vi "UI_FP size and position.vi"(4 "Close Ref? (T) In":bool=TRUE, 6 "Move Window (f) In":bool, 7 "FP Origin (0,0) In":cluster{"Horizontal":i16, "Vertical":i16}, 8 "Error In":errorcluster, 9 "Window Size(No Resize) In":cluster{"Width":i16, "Height":i16}, 10 "Window Origin (0,0) In":cluster{"Left":i16, "Top":i16}, 11 "Vi Ref (this Vi) In":refnum<vi>) -> (0 "Error Out":errorcluster, 3 "Dup Ref Out":refnum<vi>)   [LabVIEW 2009]
doc: "Sets VI Front Panel to specified position and size"
panel:
  in  "Set Values":bool
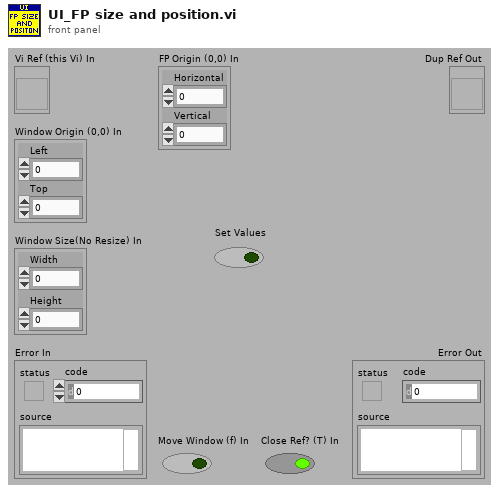
[diagram p1: front panel]
types:
  T1 = typedef "LVRectTypeDef.ctl" = cluster{"left":i16, "top":i16, "right":i16, "bottom":i16}
  T2 = typedef "LVPointTypeDef.ctl" = cluster{"Horizontal":i16, "Vertical":i16}
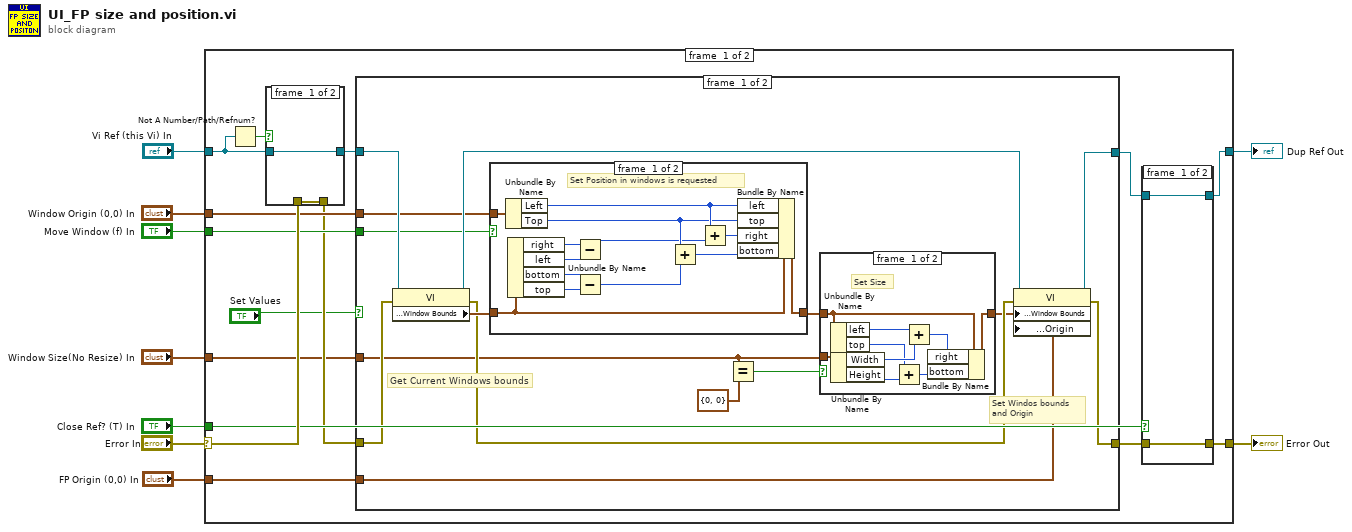
[diagram p0: block diagram]
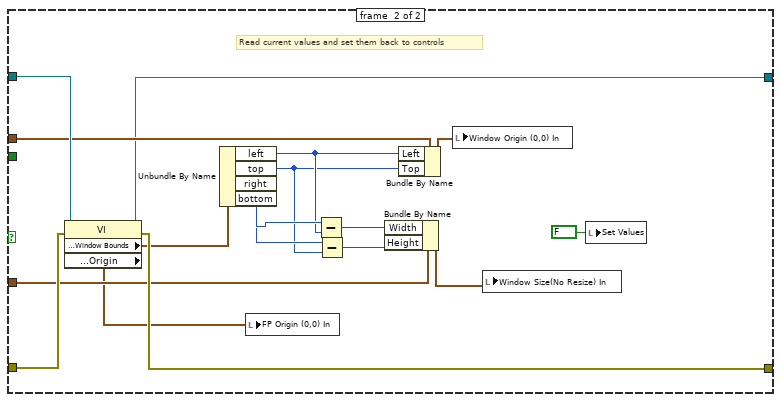
[diagram p4: hidden frame]
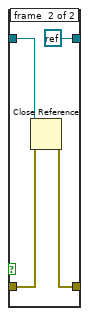
[diagram p5: hidden frame]
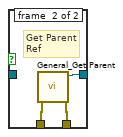
[diagram p6: hidden frame]
diagram:
  n1 = case shown="No Error" "Error In" {
    selector: "Error In" -> [w20 w92]
    tunnel: "Vi Ref (this Vi) In" -> [w21 w93]
    tunnel: [w17 w93] -> w8
    tunnel: [w19 w92] -> w7
    tunnel: "FP Origin (0,0) In" -> [w12 _]
    tunnel: "Window Size(No Resize) In" -> [w11 _]
    tunnel: "Close Ref? (T) In" -> [w18 _]
    tunnel: "Window Origin (0,0) In" -> [w16 _]
    tunnel: "Move Window (f) In" -> [w15 _]
    frame #0 {
      n2 = Not A Number/Path/Refnum?(number/path/refnum=w21) -> (NaN/Path/Refnum?=w23:bool)
      n3 = case shown="True" w23 {
        tunnel: [w88 w91] -> w22
        tunnel: w21 -> [w88 _]
        tunnel: w20 -> [w87 w90]
        tunnel: [w87 w89] -> w14
        frame #0 {
        }
        frame #1 {
          # "Get Parent\nRef"
          n4 = call "General_Get Parent.vi"("Error In (no Error)"=w90) -> ("Error Out"=w89:errorcluster, "VI Refnum Out"=w91:refnum<vi>)  [unwired: 8 in, 1 out]
        }
      }
      n5 = case shown="False" "Set Values" {
        tunnel: [w38 w65] -> w24
        tunnel: w22 -> [w37 w80]
        tunnel: w16 -> [w36 w77]
        tunnel: w15 -> [w34 _]
        tunnel: w14 -> [w32 w79]
        tunnel: [w30 w78] -> w13
        tunnel: w12 -> [w28 _]
        tunnel: w11 -> [w26 w76]
        frame #0 {
          # "Set Windos bounds\nand Origin"
          # "Get Current Windows bounds"
          n6 = property class="VI"(reference=w37, error in=w32) -> (reference out=w39:refnum<vi>, error out=w31:errorcluster, "Front Panel Window:Window Bounds"=w33:T1)
          n7 = case shown="True" w34 {
            tunnel: w36 -> [w52 _]
            tunnel: [w49 w53] -> w35
            tunnel: w33 -> [w42 w53]
            frame #0 {
              # "Set Position in windows is requested"
              n8 = Unbundle By Name(w52) -> ("Left"=w48:i16, "Top"=w47:i16)
              n9 = Unbundle By Name(w42) -> ("right"=w46:i16, "left"=w45:i16, "bottom"=w44:i16, "top"=w43:i16)
              n10 = Subtract(x=w46, y=w45) -> (x-y=w41:i16)
              n11 = Subtract(x=w44, y=w43) -> (x-y=w40:i16)
              n12 = Add(x=w47, y=w40) -> (x+y=w50:i16)
              n13 = Add(x=w48, y=w41) -> (x+y=w51:i16)
              n14 = Bundle By Name(cluster=w42, "left"=w48, "top"=w47, "right"=w51, "bottom"=w50) -> (w49:T1)
            }
            frame #1 {
            }
          }
          n15 = Equal?(x=w26, y=cluster{"Width (800)":i16, "Height (600)":i16} {"Width (800)"=0, "Height (600)"=0} ("Window Size (800,600)")) -> (x = y?=w25:bool)
          n16 = case shown="False" w25 {
            tunnel: w35 -> [w59 w63]
            tunnel: w26 -> [w62 _]
            tunnel: [w58 w63] -> w29
            frame #0 {
              # "Set Size"
              n17 = Unbundle By Name(w59) -> ("left"=w57:i16, "top"=w56:i16)
              n18 = Unbundle By Name(w62) -> ("Width"=w60:i16, "Height"=w61:i16)
              n19 = Add(x=w56, y=w61) -> (x+y=w54:i16)
              n20 = Add(x=w57, y=w60) -> (x+y=w55:i16)
              n21 = Bundle By Name(cluster=w59, "right"=w55, "bottom"=w54) -> (w58:T1)
            }
            frame #1 {
            }
          }
          n22 = property class="VI"(reference=w39, error in=w31, "Front Panel Window:Window Bounds"=w29, "Front Panel Window:Origin"=w28) -> (reference out=w38:refnum<vi>, error out=w30:errorcluster)
        }
        frame #1 {
          # "Read current values and set them back to controls"
          n23 = property class="VI"(reference=w80, error in=w79) -> (reference out=w65:refnum<vi>, error out=w78:errorcluster, "Front Panel Window:Window Bounds"=w74:T1, "Front Panel Window:Origin"=w75:T2)
          n24 = Unbundle By Name(w74) -> ("left"=w70:i16, "top"=w67:i16, "right"=w71:i16, "bottom"=w68:i16)
          n25 = local write "FP Origin (0,0) In"(w75) -> ()
          n26 = Subtract(x=w71, y=w70) -> (x-y=w69:i16)
          n27 = Subtract(x=w68, y=w67) -> (x-y=w66:i16)
          n28 = Bundle By Name(cluster=w76, "Width"=w69, "Height"=w66) -> (w72:cluster{"Width":i16, "Height":i16})
          n29 = Bundle By Name(cluster=w77, "Left"=w70, "Top"=w67) -> (w73:cluster{"Left":i16, "Top":i16})
          n30 = local write "Window Origin (0,0) In"(w73) -> ()
          n31 = local write "Window Size(No Resize) In"(w72) -> ()
          n32 = local write "Set Values"(FALSE ("Set Values")) -> ()
        }
      }
      n33 = case shown="True" w18 {
        tunnel: w24 -> [w82 w84]
        tunnel: w13 -> [w81 w86]
        tunnel: [w81 w85] -> w19
        tunnel: [w82 refnum<k0> refnum] -> w17
        frame #0 {
        }
        frame #1 {
          n34 = Close Reference(reference=w84, error in (no error)=w86) -> (error out=w85:errorcluster)
        }
      }
    }
    frame #1 {
    }
  }
  "Dup Ref Out" <- w8
  "Error Out" <- w7
